vi "Create Folder File and Contents If Not Existing.vi"(4 "error in (no error)":errorcluster, 5 "File contents to write (\"\")":string, 6 "Filename (\"\")":string, 7 "File Folder (Empty)":path) -> (0 "error out":errorcluster, 2 "Already Existed?":bool, 3 "Path to File":path)   [LabVIEW 2011]
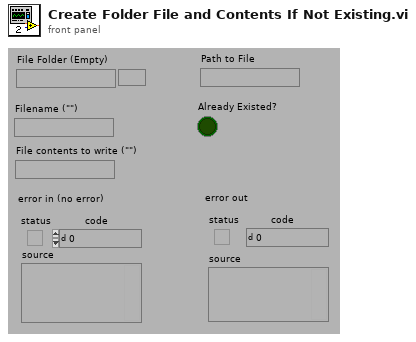
[diagram p1: front panel]
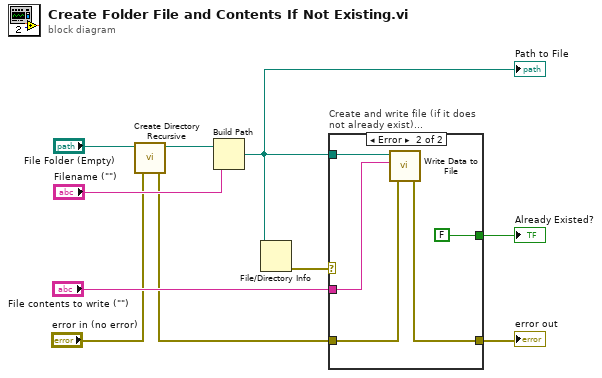
[diagram p0: block diagram]
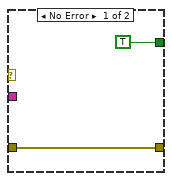
[diagram p2: hidden frame]
diagram:
  n1 = call <vilib>:"Create Directory Recursive.vi"("error in (no error)"="error in (no error)", "directory"="File Folder (Empty)") -> ("error out"=w3:errorcluster, "directory copy"=w10:path)  [unwired: 1 in, 3 out]
  n2 = Build Path(base path=w10, name or relative path="Filename (\"\")") -> (appended path=w1:path)
  "Path to File" <- w1
  n3 = File/Directory Info(path=w1) -> (error out=w5:errorcluster)  [unwired: 1 in, 6 out]
  n4 = case "Create and write file (if it does\nnot already exist)..." shown="Error" w5 {
    tunnel: w1 -> [_ w17]
    tunnel: w3 -> [w12 w15]
    tunnel: "File contents to write (\"\")" -> [_ w16]
    tunnel: [w12 w14] -> w7
    tunnel: [TRUE FALSE] -> w2
    frame No Error {
    }
    frame Error {
      n5 = call "Write Data to File.vi"("error in (no error)"=w15, "Data to Write"=w16, "File to Write"=w17) -> ("error out"=w14:errorcluster)  [unwired: 4 out]
    }
  }
  "error out" <- w7
  "Already Existed?" <- w2
